vi "DialGauge.vi"() -> ()   [LabVIEW 2024]
uses:
  <vilib>/Utility/miscctls.llb/LVRowAndColumnTypeDef.ctl
  Library/Class/Renishaw-XL80/Renishaw-XL80.lvclass
  Library/Class/Renishaw-XL80_EMU/Renishaw-XL80_EMU.lvclass
  <vilib>/Analysis/1siggen.llb/Ramp Pattern by Delta.vi
  <vilib>/Analysis/NI_AALBase.lvlib
panel:
  out "Max Any":ext
  out "Max 2.0":ext
  out "Max 1.0":ext
  out "Max 0.5":ext
  out "Max 0.1":ext
  in  "Calculate":bool
  in  "Multicolumn Listbox":i32(listbox)
  out "output cluster":cluster{"nextRow":dbl, "nextColumn":dbl}
  out "Current":T1
  out "ScanCode":i16
  in  "Table Control":string[][](table)
  out "Edit Position":T1
  out "nominal":dbl format="%.1f"
  out "Signal":dbl(slide) scale=0.0..31.0
  in  "sign_mode":bool
  out "Zero Value":dbl format="%_8f"
  out "Mat Temp":dbl[](array[numeric]) caption="Mat Temp(°C)"
  out "Air Temp":dbl caption="Air Temp(°C)"
  in  "Reset":bool
  in  "Connect":bool
  in  "Zero":bool
  out "Serial Number":string caption="Laser Device ID"
  out "Connected":bool
  in  "Precision":u16(ring)=4 items=["0 digit", "1 digit", "2 digits", "3 digits", "4 digits", "5 digits", "6 digits"]
  in  "Unit":u16(ring) caption="mm/inch" items=["mm", "inch"]
  out "Measurement":dbl format="%.3f"
  in  "Description":string
  in  "Manufacturer":string
  in  "Ref equipment ID":string
  in  "Model No.":string
  in  "S/No. or ID":string
  in  "Job No.":string
  out "uncalibrated":dbl
  out "error out":errorcluster
  in  "error IO":errorcluster
  # "Job Info"
  # "DUT Info"
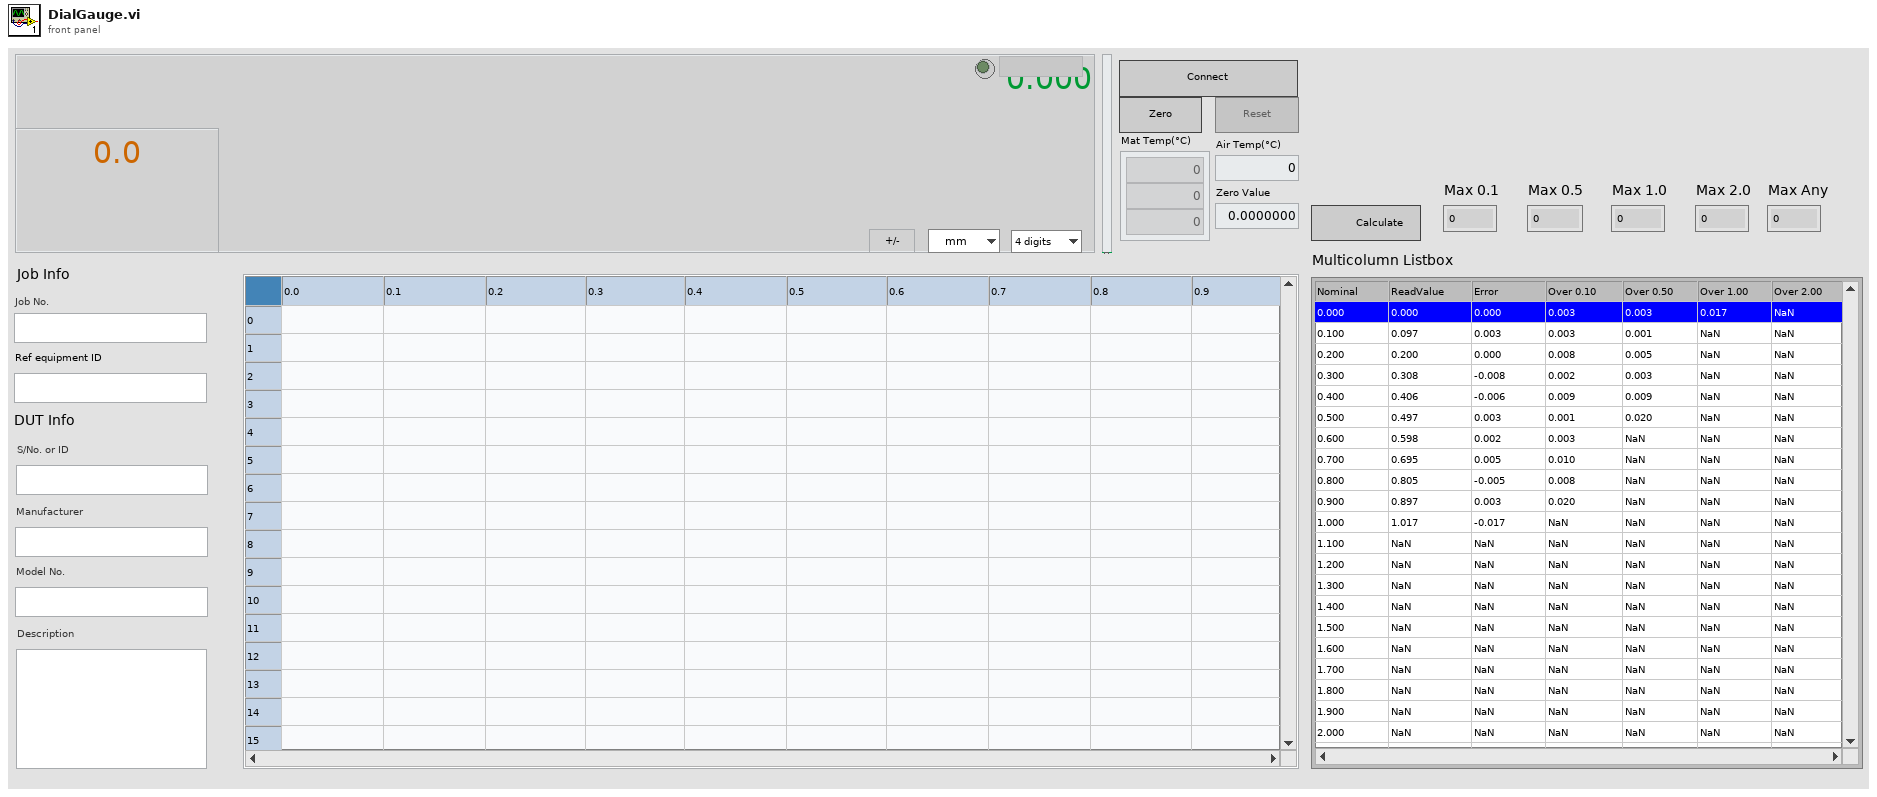
[diagram p1: front panel]
types:
  T1 = typedef "LVRowAndColumnTypeDef.ctl" = cluster{"Row":i32, "Column":i32}
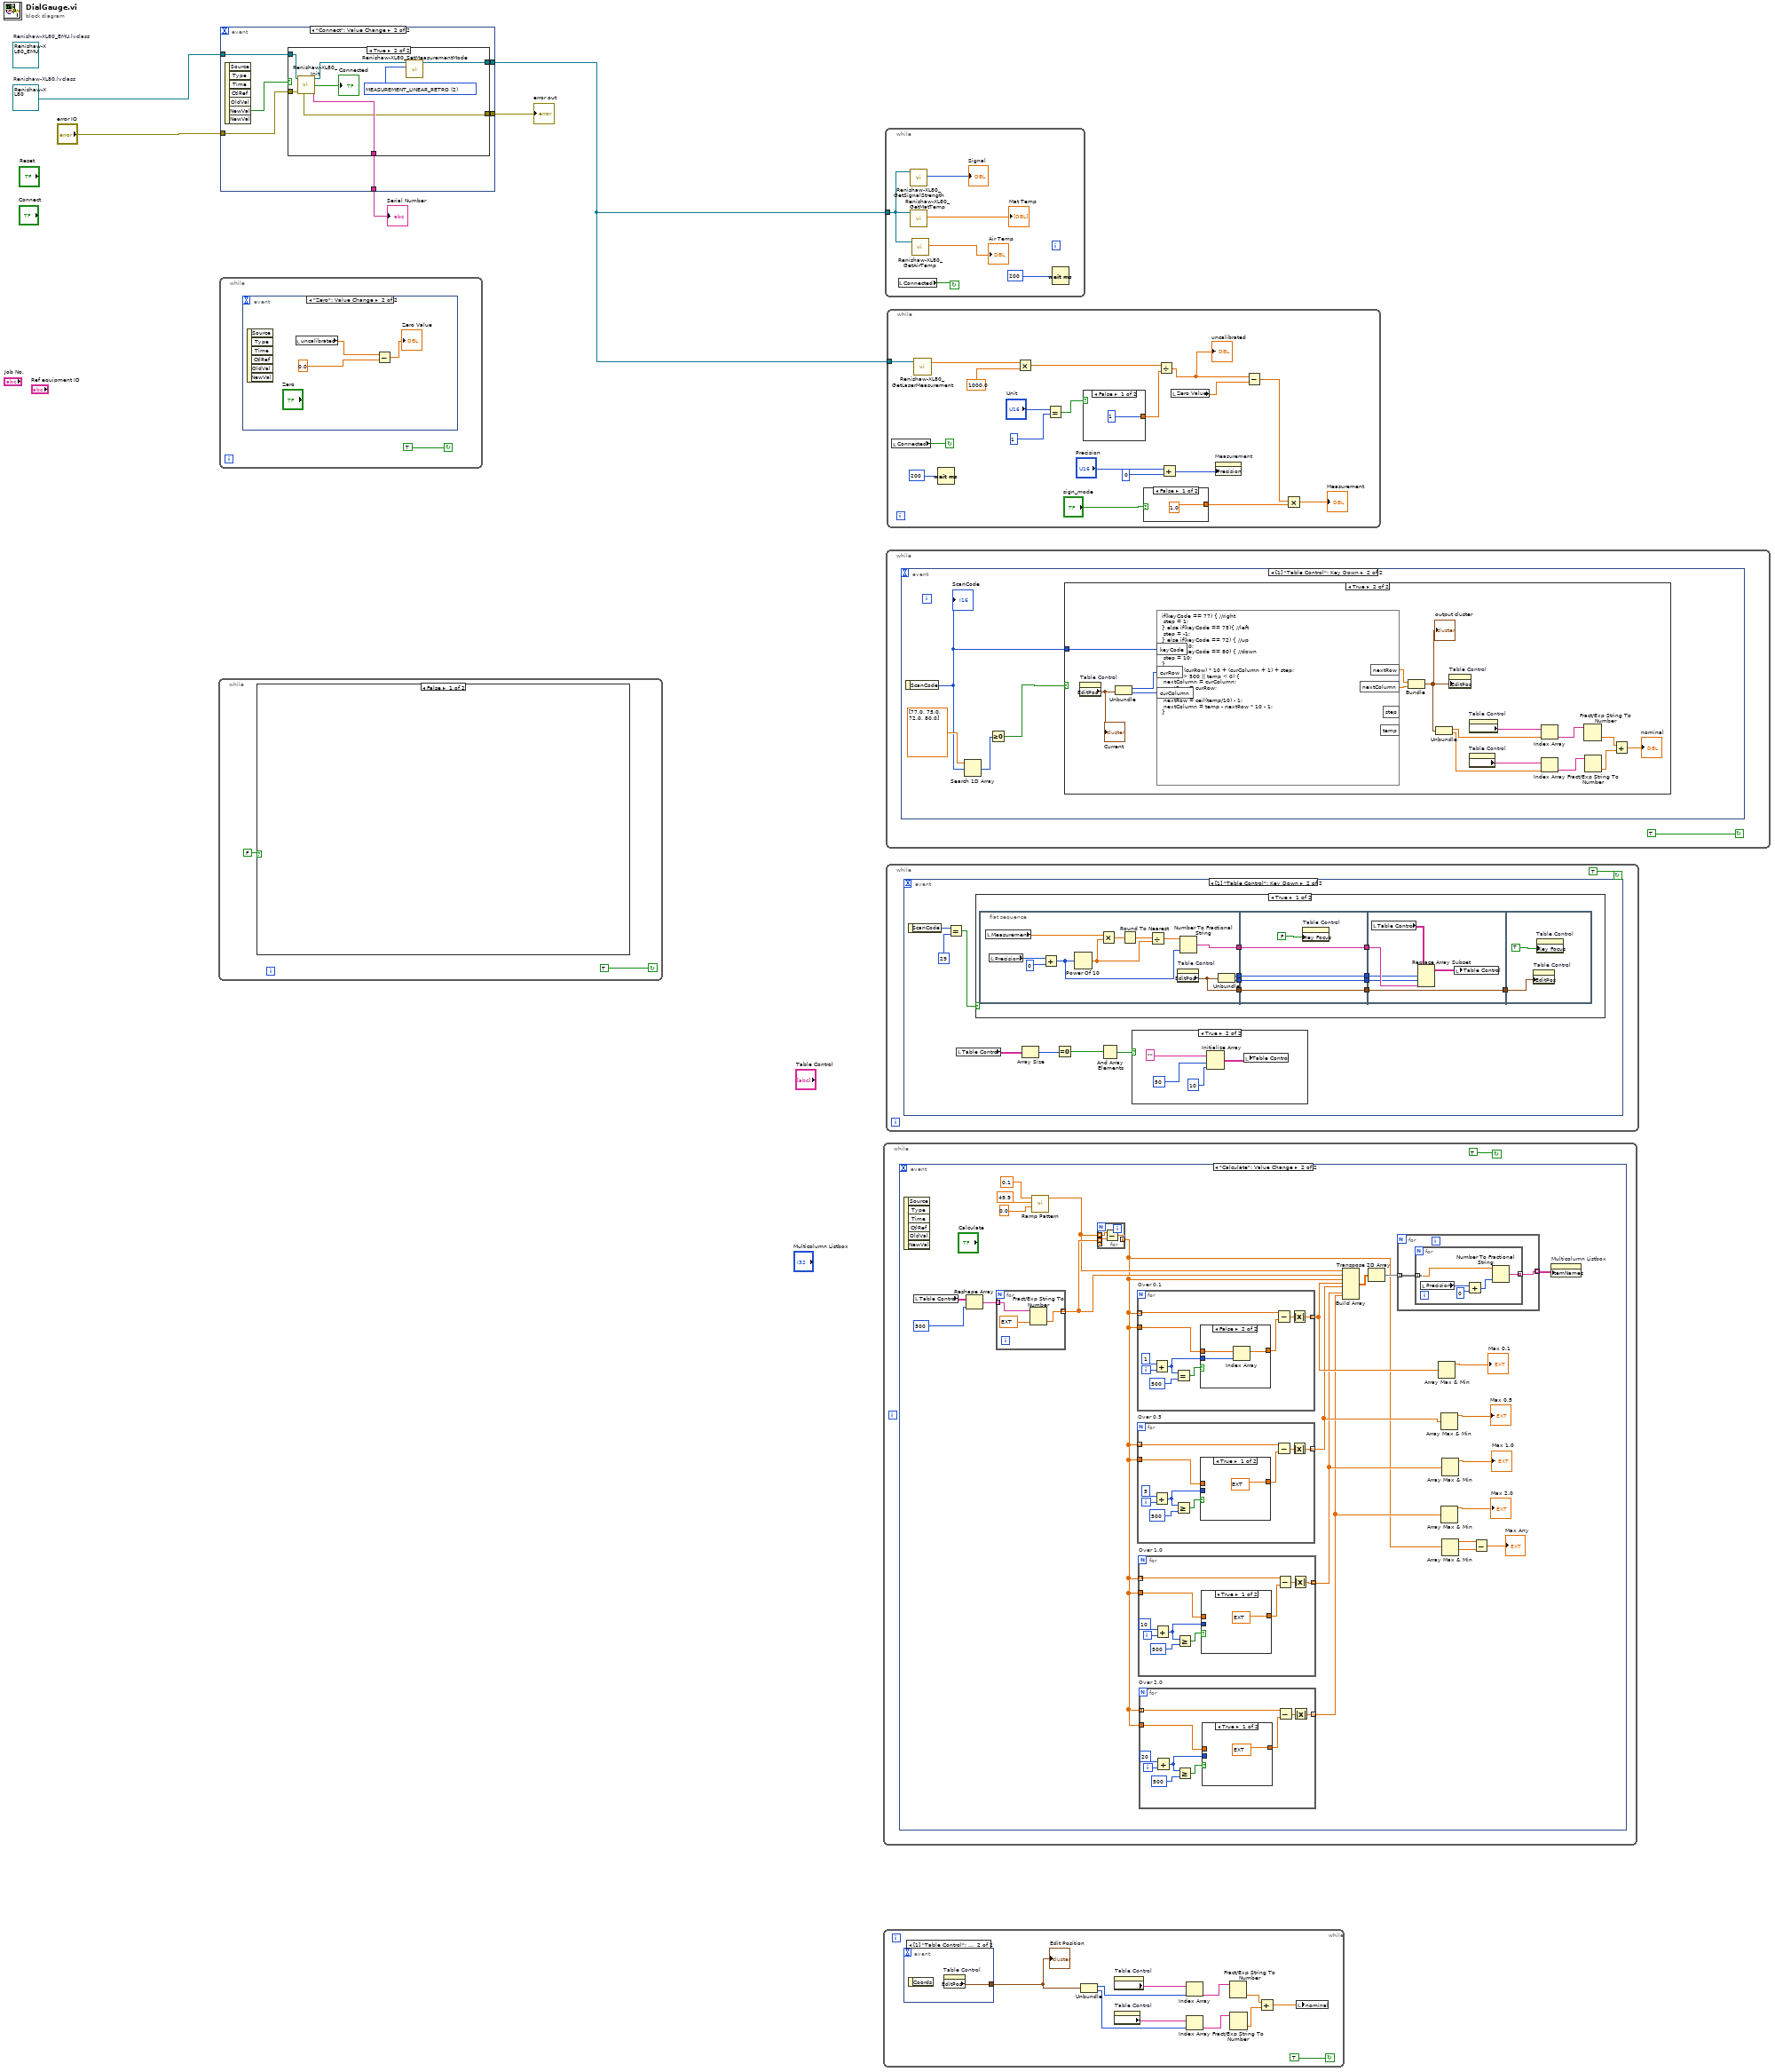
[diagram p0: block diagram]
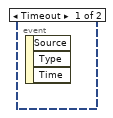
[diagram p2: hidden frame]
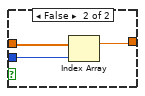
[diagram p3: hidden frame]
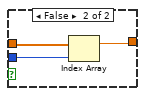
[diagram p4: hidden frame]
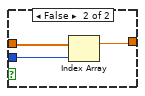
[diagram p5: hidden frame]
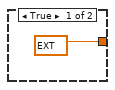
[diagram p6: hidden frame]
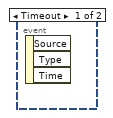
[diagram p7: hidden frame]
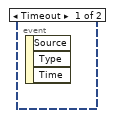
[diagram p10: hidden frame]
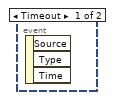
[diagram p12: hidden frame]
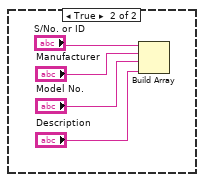
[diagram p13: hidden frame]
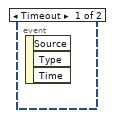
[diagram p14: hidden frame]
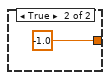
[diagram p15: hidden frame]
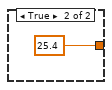
[diagram p16: hidden frame]
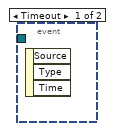
[diagram p17: hidden frame]
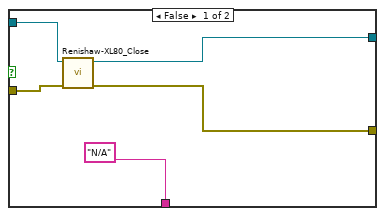
[diagram p18: hidden frame]
diagram:
  (unwired) refnum<class "Renishaw-XL80_EMU.lvclass"> refnum  # Renishaw-XL80_EMU.lvclass
  w1 = refnum<class "Renishaw-XL80.lvclass"> refnum  # Renishaw-XL80.lvclass
  n1 = while {
    stop <- TRUE continue-if-true
    n2 = case shown="False" FALSE {
      frame False {
      }
      frame True {
        n3 = Build Array("S/No. or ID", "Manufacturer", "Model No.", "Description") -> ()  [unwired: 1 out]
      }
    }
  }
  n4 = while {
    stop <- TRUE continue-if-true
    n5 = event shown="[1] \"Zero\": Value Change" {
      selector: _ -> [_ _]
      dyn-events: _ -> [_ _]
      timeout: _ -> [_ _]
      event Timeout {
        n6 = event-data() -> ()  [unwired: 1 in, 3 out]
      }
      event "Zero": Value Change {
        n7 = event-data() -> ()  [unwired: 1 in, 6 out]
        n8 = local read "uncalibrated"() -> (w15:dbl)
        n9 = Subtract(x=w15, y=0.0) -> (x-y=→"Zero Value":dbl)
      }
    }
  }
  n10 = event shown="[1] \"Connect\": Value Change" {
    selector: _ -> [_ _]
    dyn-events: _ -> [_ _]
    timeout: _ -> [_ _]
    tunnel: w1 -> [_ w21]
    tunnel: [_ w20] -> w4
    tunnel: [_ w19] -> w5
    tunnel: "error IO" -> [_ w18]
    tunnel: [_ w17] -> w3
    event Timeout {
      n11 = event-data() -> ()  [unwired: 1 in, 3 out]
    }
    event "Connect": Value Change {
      n12 = event-data() -> ("NewVal"=w16:bool)  [unwired: 1 in, 6 out]
      n13 = case shown="True" w16 {
        tunnel: w21 -> [w26 w34]
        tunnel: ["N/A" ("Serial Number") w33] -> w19
        tunnel: [w25 w28] -> w20
        tunnel: w18 -> [w24 w32]
        tunnel: [w23 w31] -> w17
        frame False {
          n14 = call-dynamic "Renishaw-XL80_Close.vi"("error in (no error)"=w24, "Renishaw-XL80 in"=w26) -> ("error out"=w23:errorcluster, "Renishaw-XL80 out"=w25:refnum<class "Renishaw-XL80.lvclass">)  [unwired: 8 in]
        }
        frame True {
          w27 = 2 items=["MEASUREMENT_INDETERMINATE", "MEASUREMENT_LINEAR_PLANE", "MEASUREMENT_LINEAR_RETRO", "MEASUREMENT_ANGULAR", "MEASUREMENT_STRAIGHTNESS_SHORT", "MEASUREMENT_STRAIGHTNESS_LONG", "MEASUREMENT_VELOCITY_RETRO"] ("MeasurementMode")
          n15 = call-dynamic "Renishaw-XL80_Init.vi"("error in (no error)"=w32, "Renishaw-XL80 in"=w34) -> ("error out"=w31:errorcluster, "Serial Number"=w33:string, "Connect"=→"Connected":bool, "Renishaw-XL80 out"=w29:refnum<class "Renishaw-XL80.lvclass">)  [unwired: 6 in]
          n16 = call-dynamic "Renishaw-XL80_SetMeasurementMode.vi"("MeasurementMode"=w27, "Renishaw-XL80 in"=w29) -> ("Renishaw-XL80 out"=w28:refnum<class "Renishaw-XL80.lvclass">)  [unwired: 8 in, 1 out]
        }
      }
    }
  }
  "error out" <- w3
  "Serial Number" <- w5
  n17 = while {
    stop <- TRUE continue-if-true
    n18 = event shown="[1] \"Calculate\": Value Change" {
      selector: _ -> [_ _]
      dyn-events: _ -> [_ _]
      timeout: _ -> [_ _]
      event Timeout {
        n19 = event-data() -> ()  [unwired: 1 in, 3 out]
      }
      event "Calculate": Value Change {
        n20 = event-data() -> ()  [unwired: 1 in, 6 out]
        n21 = local read "Table Control"() -> (w58:string[][])
        n22 = Reshape Array(w58, 500 ("dimension size")) -> (w52:string[])
        n23 = for {
          tunnel: w52 -> [w126] mode=indexing
          tunnel: [w127] -> w49 mode=indexing
          n24 = Fract/Exp String To Number(string=w126, default (0 dbl)=ext nan ("default (0 DBL)")) -> (number=w127:ext)  [unwired: 2 in, 1 out]
        }
        n25 = call-poly <vilib>:"Ramp Pattern.vi"("start"=0.0, "end"=49.9, "delta"=0.1) -> ("Ramp Pattern"=w48:dbl[])  [unwired: 6 in, 2 out]
        n26 = for {
          tunnel: [w116] -> _ mode=indexing
          tunnel: w49 -> [w116] mode=indexing
          tunnel: w48 -> [w117] mode=indexing
          tunnel: [w115] -> w39 mode=indexing
          n27 = Subtract(x=w117, y=w116) -> (x-y=w115:ext)
        }
        n28 = for "Over 0.1" {
          tunnel: w39 -> [w108] mode=indexing
          tunnel: w39 -> [w105]
          tunnel: [w106] -> w46 mode=indexing
          i -> [w110]
          n29 = Add(x=1, y=w110) -> (x+y=w101:i32)
          n30 = Equal?(x=w101, y=500) -> (x = y?=w102:bool)
          n31 = case shown="False" w102 {
            tunnel: w105 -> [_ w114]
            tunnel: [ext nan w113] -> w104
            tunnel: w101 -> [_ w112]
            frame True {
            }
            frame False {
              n32 = Index Array(array=w114, index=w112) -> (element=w113:ext)
            }
          }
          n33 = Subtract(x=w108, y=w104) -> (x-y=w107:ext)
          n34 = Absolute Value(x=w107) -> (abs(x)=w106:ext)
        }
        n35 = for "Over 0.5" {
          tunnel: w39 -> [w94] mode=indexing
          tunnel: w39 -> [w91]
          tunnel: [w92] -> w42 mode=indexing
          i -> [w96]
          n36 = Add(x=5, y=w96) -> (x+y=w87:i32)
          n37 = Greater Or Equal?(x=w87, y=500) -> (x >= y?=w88:bool)
          n38 = case shown="True" w88 {
            tunnel: w91 -> [_ w100]
            tunnel: [ext nan w99] -> w90
            tunnel: w87 -> [_ w98]
            frame True {
            }
            frame False {
              n39 = Index Array(array=w100, index=w98) -> (element=w99:ext)
            }
          }
          n40 = Subtract(x=w94, y=w90) -> (x-y=w93:ext)
          n41 = Absolute Value(x=w93) -> (abs(x)=w92:ext)
        }
        n42 = for "Over 1.0" {
          tunnel: w39 -> [w80] mode=indexing
          tunnel: w39 -> [w77]
          tunnel: [w78] -> w41 mode=indexing
          i -> [w82]
          n43 = Add(x=10, y=w82) -> (x+y=w73:i32)
          n44 = Greater Or Equal?(x=w73, y=500) -> (x >= y?=w74:bool)
          n45 = case shown="True" w74 {
            tunnel: w77 -> [_ w86]
            tunnel: [ext nan w85] -> w76
            tunnel: w73 -> [_ w84]
            frame True {
            }
            frame False {
              n46 = Index Array(array=w86, index=w84) -> (element=w85:ext)
            }
          }
          n47 = Subtract(x=w80, y=w76) -> (x-y=w79:ext)
          n48 = Absolute Value(x=w79) -> (abs(x)=w78:ext)
        }
        n49 = for "Over 2.0" {
          tunnel: w39 -> [w66] mode=indexing
          tunnel: w39 -> [w63]
          tunnel: [w64] -> w40 mode=indexing
          i -> [w68]
          n50 = Add(x=20, y=w68) -> (x+y=w59:i32)
          n51 = Greater Or Equal?(x=w59, y=500) -> (x >= y?=w60:bool)
          n52 = case shown="True" w60 {
            tunnel: w63 -> [_ w72]
            tunnel: [ext nan w71] -> w62
            tunnel: w59 -> [_ w70]
            frame True {
            }
            frame False {
              n53 = Index Array(array=w72, index=w70) -> (element=w71:ext)
            }
          }
          n54 = Subtract(x=w66, y=w62) -> (x-y=w65:ext)
          n55 = Absolute Value(x=w65) -> (abs(x)=w64:ext)
        }
        n56 = Build Array(w48, w49, w39, w46, w42, w41, w40) -> (w56:ext[][])
        n57 = Transpose 2D Array(2D array=w56) -> (transposed array=w51:ext[][])
        n58 = for {
          tunnel: w51 -> [w119] mode=indexing
          tunnel: [w118] -> w50 mode=indexing
          n59 = for {
            tunnel: w119 -> [w122] mode=indexing
            tunnel: [w120] -> w118 mode=indexing
            n60 = local read "Precision"() -> (w123:u16)
            n61 = Add(x=w123, y=u16 0) -> (x+y=w121:u16)
            n62 = Number To Fractional String(number=w122, precision (6)=w121) -> (F-format string=w120:string)  [unwired: 2 in]
          }
        }
        n63 = Array Max & Min(array=w46) -> (max value=→"Max 0.1":ext)  [unwired: 3 out]
        n64 = Array Max & Min(array=w42) -> (max value=→"Max 0.5":ext)  [unwired: 3 out]
        n65 = Array Max & Min(array=w40) -> (max value=→"Max 2.0":ext)  [unwired: 3 out]
        n66 = Array Max & Min(array=w41) -> (max value=→"Max 1.0":ext)  [unwired: 3 out]
        n67 = Array Max & Min(array=w39) -> (max value=w38:ext, min value=w37:ext)  [unwired: 2 out]
        n68 = Subtract(x=w38, y=w37) -> (x-y=→"Max Any":ext)
        n69 = property on="Multicolumn Listbox" class="MCListbox (strict)"("ItemNames"=w50) -> ()  [unwired: 2 in, 2 out]
      }
    }
  }
  n70 = while {
    stop <- TRUE continue-if-true
    n71 = event shown="[1] \"Table Control\": Mouse Down" {
      selector: _ -> [_ _]
      dyn-events: _ -> [_ _]
      timeout: _ -> [_ _]
      tunnel: [_ w139] -> w129
      event Timeout {
        n72 = event-data() -> ()  [unwired: 1 in, 3 out]
      }
      event "Table Control": Mouse Down {
        n73 = event-data() -> ()  [unwired: 1 in, 1 out]
        n74 = property on="Table Control" class="Tbl (strict)"() -> ("EditPos"=w139:T1)  [unwired: 2 in, 2 out]
      }
    }
    "Edit Position" <- w129
    n75 = Unbundle(w129) -> ("Row"=w131:i32, "Column"=w137:i32)
    n76 = property on="Table Control" class="Tbl (strict)"() -> ("Row Headers[]"=w130:string[])  [unwired: 2 in, 2 out]
    n77 = property on="Table Control" class="Tbl (strict)"() -> ("Column Headers[]"=w132:string[])  [unwired: 2 in, 2 out]
    n78 = Index Array(array=w130, index=w131) -> (element=w133:string)
    n79 = Index Array(array=w132, index=w137) -> (element=w134:string)
    n80 = Fract/Exp String To Number(string=w133) -> (number=w135:dbl)  [unwired: 3 in, 1 out]
    n81 = Fract/Exp String To Number(string=w134) -> (number=w136:dbl)  [unwired: 3 in, 1 out]
    n82 = Add(x=w135, y=w136) -> (x+y=w128:dbl)
    n83 = local write "nominal"(w128) -> ()
  }
  n84 = while {
    tunnel: w4 -> [w141]
    stop <- w142 continue-if-true
    n85 = local read "Connected"() -> (w142:bool)
    n86 = call-dynamic "Renishaw-XL80_GetSignalStrength.vi"("Renishaw-XL80 in"=w141) -> ("Signal Strength"=→"Signal":i16)  [unwired: 8 in, 2 out]
    n87 = call-dynamic "Renishaw-XL80_GetMatTemp.vi"("Renishaw-XL80 in"=w141) -> ("Temperature Array"=→"Mat Temp":dbl[])  [unwired: 7 in, 3 out]
    n88 = call-dynamic "Renishaw-XL80_GetAirTemp.vi"("Renishaw-XL80 in"=w141) -> ("GetAirTemp"=→"Air Temp":dbl)  [unwired: 7 in, 3 out]
    n89 = Wait (ms)(milliseconds to wait=u32 200) -> ()  [unwired: 1 out]
  }
  n90 = while {
    stop <- TRUE continue-if-true
    n91 = event shown="[1] \"Table Control\": Key Down" {
      selector: _ -> [_ _]
      dyn-events: _ -> [_ _]
      timeout: _ -> [_ _]
      event Timeout {
        n92 = event-data() -> ()  [unwired: 1 in, 3 out]
      }
      event "Table Control": Key Down {
        n93 = event-data() -> ("ScanCode"=w147:i16)  [unwired: 1 in]
        "ScanCode" <- w147
        n94 = Search 1D Array(1D array=dbl[] [77.0, 75.0, 72.0, 80.0], element=w147) -> (index of element=w149:i32)  [unwired: 1 in]
        n95 = Greater Or Equal To 0?(x=w149) -> (x >= 0?=w148:bool)
        n96 = case shown="True" w148 {
          tunnel: w147 -> [_ w166]
          frame False {
          }
          frame True {
            n97 = property on="Table Control" class="Tbl (strict)"() -> ("EditPos"=w161:T1)  [unwired: 2 in, 2 out]
            "Current" <- w161
            n98 = Unbundle(w161) -> ("Row"=w165:i32, "Column"=w164:i32)
            n99 = formula code="if(keyCode == 77) { //right\n\tstep = 1;\n} else if(keyCode == 75){ //left\n\tstep = -1;\n} else if(keyCode == 72) { //up\n\tstep = -10;\n} else if(keyCode == 80) { //down\n\tstep = 10;\n}\ntemp = (curRow) * 10 + (curColumn + 1) + step;\nif(temp > 500 || temp < 0) {\n\tnextColumn = curColumn;\n\tnextRow = curRow;\n} else {\n\tnextRow = ceil(temp/10) - 1;\n\tnextColumn = temp - nextRow * 10 - 1;\n}"("keyCode"=w166, "curRow"=w165, "curColumn"=w164) -> ("nextRow"=w163:dbl, "nextColumn"=w162:dbl)  [unwired: 2 out]
            n100 = Bundle("nextRow"=w163, "nextColumn"=w162) -> (w151:cluster{"nextRow":dbl, "nextColumn":dbl})  [unwired: 1 in]
            "output cluster" <- w151
            n101 = Unbundle(w151) -> ("nextRow"=w159:dbl, "nextColumn"=w152:dbl)
            n102 = property on="Table Control" class="Tbl (strict)"("EditPos"=w151) -> ()  [unwired: 2 in, 2 out]
            n103 = property on="Table Control" class="Tbl (strict)"() -> ("Row Headers[]"=w160:string[])  [unwired: 2 in, 2 out]
            n104 = property on="Table Control" class="Tbl (strict)"() -> ("Column Headers[]"=w158:string[])  [unwired: 2 in, 2 out]
            n105 = Index Array(array=w160, index=w159) -> (element=w157:string)
            n106 = Index Array(array=w158, index=w152) -> (element=w156:string)
            n107 = Fract/Exp String To Number(string=w157) -> (number=w155:dbl)  [unwired: 3 in, 1 out]
            n108 = Fract/Exp String To Number(string=w156) -> (number=w154:dbl)  [unwired: 3 in, 1 out]
            n109 = Add(x=w155, y=w154) -> (x+y=→"nominal":dbl)
          }
        }
      }
    }
  }
  n110 = while {
    stop <- TRUE continue-if-true
    n111 = event shown="[1] \"Table Control\": Key Down" {
      selector: _ -> [_ _]
      dyn-events: _ -> [_ _]
      timeout: _ -> [_ _]
      event Timeout {
        n112 = event-data() -> ()  [unwired: 1 in, 3 out]
      }
      event "Table Control": Key Down {
        n113 = event-data() -> ("ScanCode"=w173:i16)  [unwired: 1 in]
        n114 = Equal?(x=w173, y=i16 29) -> (x = y?=w172:bool)
        n115 = local read "Table Control"() -> (w171:string[][])
        n116 = case shown="True" w172 {
          frame True {
            n117 = flat-sequence {
              tunnel: [w191] -> w187
              tunnel: [w190] -> w184
              tunnel: [w189] -> w182
              tunnel: [w188] -> w179
              tunnel: w187 -> [w204]
              tunnel: [w204] -> w186
              tunnel: [w202] -> w185
              tunnel: w184 -> [w202]
              tunnel: [w201] -> w183
              tunnel: w182 -> [w201]
              tunnel: [w200] -> w180
              tunnel: w179 -> [w200]
              tunnel: w186 -> [w209]
              tunnel: w185 -> [w208]
              tunnel: w183 -> [w207]
              tunnel: [w205] -> w181
              tunnel: w180 -> [w205]
              tunnel: w181 -> [w212]
              frame #0 {
                n118 = local read "Measurement"() -> (w196:dbl)
                n119 = local read "Precision"() -> (w195:u16)
                n120 = Add(x=w195, y=u16 0) -> (x+y=w193:u16)
                n121 = Power Of 10(x=w193) -> (10^x=w199:dbl)
                n122 = Multiply(x=w196, y=w199) -> (x*y=w197:dbl)
                n123 = Round To Nearest(number=w197) -> (nearest integer value=w198:dbl)
                n124 = Divide(x=w198, y=w199) -> (x/y=w192:dbl)
                n125 = property on="Table Control" class="Tbl (strict)"() -> ("EditPos"=w188:T1)  [unwired: 2 in, 2 out]
                n126 = Number To Fractional String(number=w192, precision (6)=w193) -> (F-format string=w191:string)  [unwired: 2 in]
                n127 = Unbundle(w188) -> ("Row"=w190:i32, "Column"=w189:i32)
              }
              frame #1 {
                n128 = property on="Table Control" class="Tbl (strict)"("Key Focus"=FALSE) -> ()  [unwired: 2 in, 2 out]
              }
              frame #2 {
                n129 = local read "Table Control"() -> (w210:string[][])
                n130 = Replace Array Subset(array=w210, new element=w209, index (row)=w208, index (col)=w207) -> (w206:string[][])
                n131 = local write "Table Control"(w206) -> ()
              }
              frame #3 {
                n132 = property on="Table Control" class="Tbl (strict)"("EditPos"=w212) -> ()  [unwired: 2 in, 2 out]
                n133 = property on="Table Control" class="Tbl (strict)"("Key Focus"=TRUE) -> ()  [unwired: 2 in, 2 out]
              }
            }
          }
          frame False {
          }
        }
        n134 = Array Size(array=w171) -> (size(s)=w170:i32[])
        n135 = Equal To 0?(x=w170) -> (x = 0?=w169:bool[])
        n136 = And Array Elements(Boolean array=w169) -> (logical AND=w168:bool)
        n137 = case shown="True" w168 {
          frame False {
          }
          frame True {
            n138 = Initialize Array("", 50 ("dimension size"), 10 ("dimension size")) -> (w178:string[][])
            n139 = local write "Table Control"(w178) -> ()
          }
        }
      }
    }
  }
  n140 = while {
    tunnel: w4 -> [w231]
    stop <- w220 continue-if-true
    n141 = local read "Connected"() -> (w220:bool)
    n142 = call-dynamic "Renishaw-XL80_GetLaserMeasurement.vi"("Renishaw-XL80 in"=w231) -> ("GetLaserMeasurement"=w229:dbl)  [unwired: 7 in, 3 out]
    n143 = Wait (ms)(milliseconds to wait=u32 200) -> ()  [unwired: 1 out]
    n144 = Multiply(x=w229, y=1000.0) -> (x*y=w221:dbl)
    n145 = Equal?(x="Unit", y=u16 1) -> (x = y?=w223:bool)
    n146 = case shown="False" w223 {
      tunnel: [1 25.4] -> w222
      frame False {
      }
      frame True {
      }
    }
    n147 = case shown="False" "sign_mode" {
      tunnel: [1.0 -1.0] -> w215
      frame False {
      }
      frame True {
      }
    }
    n148 = Divide(x=w221, y=w222) -> (x/y=w218:dbl)
    "uncalibrated" <- w218
    n149 = Add(x="Precision", y=u16 0) -> (x+y=w217:u16)
    n150 = local read "Zero Value"() -> (w219:dbl)
    n151 = property on="Measurement" class="DigNum (strict)"("Precision"=w217) -> ()  [unwired: 2 in, 2 out]
    n152 = Subtract(x=w218, y=w219) -> (x-y=w214:dbl)
    n153 = Multiply(x=w214, y=w215) -> (x*y=→"Measurement":dbl)
  }
